vi "UHR-Fleezers Control (host) - 12.1.vi"() -> ()   [LabVIEW 2012] (continued)
                n291 = Divide "Y half step offset"(x=w520, y=2.0) -> (x/y=w534:dbl)
                n292 = Divide "X pix/step"(x=w522, y=w525) -> (x/y=w531:dbl)
                n293 = Negate(x=w534) -> (-x=w535:dbl)
                n294 = local read "Initial Y"() -> (w541:dbl)
                n295 = Multiply(x=w523, y=w532) -> (x*y=w542:dbl)
                n296 = Divide "X half step offset"(x=w520, y=2.0) -> (x/y=w528:dbl)
                n297 = Divide "X V/pix"(x=w520, y=w531) -> (x/y=w530:dbl)
                n298 = Multiply(x=w520, y=w525) -> (x*y=w537:dbl)
                n299 = Compound Arithmetic op=ADD(w535, w542, w541) -> (w512:dbl)
                "Pointer Y (V)" <- w512
                n300 = Multiply(x=w530, y=w524) -> (x*y=w539:dbl)
                n301 = Negate(x=w528) -> (-x=w527:dbl)
                n302 = local read "Initial X"() -> (w540:dbl)
                n303 = Negate(x=w539) -> (-x=w538:dbl)
                n304 = Compound Arithmetic op=ADD(w527, w537, w540, w538) -> (w513:dbl)
                "Pointer X (V)" <- w513
                n305 = case shown="True" "Set High F Confocal Spot (X-Y)" {
                  tunnel: w513 -> [_ w543]
                  tunnel: w512 -> [_ w544]
                  frame False {
                  }
                  frame True {
                    "Confocal Y 2 (V)" <- w544
                    "Confocal X 2 (V)" <- w543
                  }
                }
                n306 = Or(x="Set X Only", y="Set Confocal Spot (X-Y)") -> (x .or. y?=w516:bool)
                n307 = Or(x="Set Confocal Spot (X-Y)", y="Set Y Only") -> (x .or. y?=w515:bool)
                n308 = case shown="True" w516 {
                  tunnel: w513 -> [_ w545]
                  frame False {
                  }
                  frame True {
                    n309 = property on="AO2" class="Slide (strict)"("Val(Sgnl)"=w545) -> ()  [unwired: 2 in, 2 out]
                    "Confocal X 1 (V)" <- w545
                  }
                }
                n310 = case shown="True" w515 {
                  tunnel: w512 -> [_ w546]
                  frame False {
                  }
                  frame True {
                    n311 = property on="AO1" class="Slide (strict)"("Val(Sgnl)"=w546) -> ()  [unwired: 2 in, 2 out]
                    "Confocal Y 1 (V)" <- w546
                  }
                }
                n312 = local write "Set High F Confocal Spot (X-Y)"(w511) -> ()
                n313 = local write "Set Confocal Spot (X-Y)"(w511) -> ()
                n314 = local write "Set X Only"(w511) -> ()
                n315 = local write "Set Y Only"(w511) -> ()
              }
            }
          }
          frame 3 {
            n316 = local read "BD 2 Frequency 1 (MHz)"() -> (w547:dbl)
            n317 = local read "BD 1 Frequency 1 (MHz)"() -> (w548:dbl)
            n318 = local write "Manipulating Trap"(TRUE ("Manipulating Trap")) -> ()
            n319 = local write "Coords"(T7 {"Horizontal"=0, "Vertical"=0} ("Coords")) -> ()
            n320 = while {
              tunnel: w553 -> [w558]
              tunnel: w551 -> [w557]
              tunnel: w549 -> [w556]
              tunnel: w548 -> [w555]
              tunnel: w547 -> [w554]
              stop <- w559 stop-if-true
              n321 = event shown="[0] \"Pane\": Mouse Move" {
                selector: _ -> [_ _]
                dyn-events: _ -> [_ _]
                timeout: _ -> [_ _]
                tunnel: ["Force Manip Abort" w623] -> w559
                tunnel: w558 -> [w566 _]
                tunnel: w557 -> [w564 _]
                tunnel: w556 -> [w563 _]
                tunnel: w555 -> [w562 _]
                tunnel: w554 -> [w561 _]
                event Mouse Move {
                  n322 = event-data() -> ("Time"=w567:u32, "Coords"=w568:T7)  [unwired: 3 out]
                  n323 = Less?(x=w567, y=w566) -> (x < y?=w565:bool)
                  n324 = case "Makes sure old motion events prior to mouse click aren't used" shown="False" w565 {
                    tunnel: w568 -> [w610 _]
                    tunnel: w564 -> [w611 _]
                    tunnel: w563 -> [w588 _]
                    tunnel: w562 -> [w584 _]
                    tunnel: w561 -> [w583 _]
                    frame False {
                      n325 = Subtract(x=w610, y=w611) -> (x-y=w609:T7)
                      "Coords" <- w609
                      n326 = local read "Y RF Frequency Limits (MHz)"() -> (w569:T15)
                      n327 = To Double Precision Float(number=w609) -> (double precision float=w608:cluster{"Horizontal":dbl, "Vertical":dbl})
                      n328 = Multiply(x=cluster{"Horizontal":dbl, "Vertical":dbl} {"Horizontal"=-1.0, "Vertical"=1.0}, y="Manipulation Scaling") -> (x*y=w604:cluster{"Horizontal":dbl, "Vertical":dbl})
                      n329 = local read "X RF Frequency Limits (MHz)"() -> (w570:T15)
                      n330 = Multiply(x=w608, y=w604) -> (x*y=w606:cluster{"Horizontal":dbl, "Vertical":dbl})
                      n331 = Unbundle By Name(w606) -> ("Horizontal"=w601:dbl, "Vertical"=w605:dbl)
                      n332 = Unbundle By Name(w569) -> ("Maximum"=w572:dbl, "Minimum"=w571:dbl)
                      n333 = Boolean To (0,1)(Boolean="Manip. X?") -> (0, 1=w599:i16)
                      n334 = Boolean To (0,1)(Boolean="Manip. Y?") -> (0, 1=w596:i16)
                      n335 = local read "BD 1 Frequency 2 (MHz)"() -> (w586:dbl)
                      n336 = Multiply(x=w605, y=w596) -> (x*y=w598:dbl)
                      n337 = Multiply(x=w599, y=w601) -> (x*y=w602:dbl)
                      n338 = local read "BD 2 Frequency 2 (MHz)"() -> (w585:dbl)
                      n339 = Unbundle By Name(w570) -> ("Maximum"=w574:dbl, "Minimum"=w573:dbl)
                      n340 = Add(x=w583, y=w598) -> (x+y=w576:dbl)
                      n341 = Add(x=w584, y=w602) -> (x+y=w578:dbl)
                      n342 = In Range and Coerce(upper limit=w574, x=w578, lower limit=w573) -> (coerced(x)=w577:dbl)  [unwired: 1 out]
                      n343 = In Range and Coerce(upper limit=w572, x=w576, lower limit=w571) -> (coerced(x)=w575:dbl)  [unwired: 1 out]
                      n344 = Subtract(x=w577, y=w586) -> (x-y=w595:dbl)
                      n345 = Subtract(x=w575, y=w585) -> (x-y=w594:dbl)
                      n346 = Square(x=w595) -> (x^2=w593:dbl)
                      n347 = Square(x=w594) -> (x^2=w592:dbl)
                      n348 = Add(x=w593, y=w592) -> (x+y=w591:dbl)
                      n349 = Square Root(x=w591) -> (sqrt(x)=w587:dbl)
                      n350 = In Range and Coerce(upper limit="Limit Max (MHz)", x=w587, lower limit="Limit Min (MHz)") -> (In Range?=w580:bool)  [unwired: 1 out]
                      n351 = Not(x="Limits Enable") -> (.not. x?=w579:bool)
                      n352 = Or(x=w580, y=w579) -> (x .or. y?=w581:bool)
                      n353 = case shown="True" w581 {
                        tunnel: w588 -> [_ w621]
                        tunnel: w587 -> [_ w612]
                        tunnel: w577 -> [_ w619]
                        tunnel: w586 -> [_ w618]
                        tunnel: w575 -> [_ w617]
                        tunnel: w585 -> [_ w616]
                        tunnel: w570 -> [_ w614]
                        tunnel: w569 -> [_ w613]
                        frame False {
                        }
                        frame True {
                          n354 = local read "BD 1 Frequency 3 (MHz)"() -> (w620:dbl)
                          n355 = local read "BD 2 Frequency 3 (MHz)"() -> (w615:dbl)
                          n356 = local write "Trap Delta (MHz)"(w612) -> ()
                          n357 = call "set RF board frequency - interlace.vi"("Board 2 Frequency Limits"=w613, "Board 1 Frequency Limits"=w614, "FPGA VI Reference In"=w621, "Board 2 Frequency 3 (MHz)"=w615, "Board 1 Frequency 3 (MHz)"=w620, "Board 2 Frequency 2 (MHz)"=w616, "Board 2 Frequency 1 (MHz)"=w617, "Board 1 Frequency 2 (MHz)"=w618, "Board 1 Frequency 1  (MHz)"=w619) -> ()  [unwired: 1 in, 2 out]
                          n358 = local write "BD 2 Frequency 1 (MHz)"(w617) -> ()
                          n359 = local write "BD 1 Frequency 1 (MHz)"(w619) -> ()
                        }
                      }
                    }
                    frame True {
                    }
                  }
                }
                event Mouse Up {
                  n360 = event-data() -> ("Button"=w622:u16)  [unwired: 8 out]
                  n361 = case shown="3" w622 {
                    tunnel: [FALSE TRUE] -> w623
                    frame 0, Default {
                    }
                    frame 3 {
                      n362 = local read "Trap Delta (MHz)"() -> (w625:dbl)
                      n363 = property on="Initial delta (MHz)" class="DigNum (strict)"("Val(Sgnl)"=w625) -> ()  [unwired: 2 in, 2 out]
                      n364 = local write "Manipulating Trap"(FALSE ("Manipulating Trap")) -> ()
                    }
                  }
                }
              }
            }
          }
        }
      }
      event Mouse Move {
        n365 = event-data() -> ()  [unwired: 6 out]
      }
    }
    n366 = local read "Stop All"() -> (w441:bool)
    n367 = node-c288() -> ()  [unwired: 2 out]
  }
  n368 = timed-loop "Run Scripts, including: stage motion" {
    tunnel: w108 -> [w634]
    tunnel: w107 -> [w635]
    tunnel: [w635] -> w106
    tunnel: [w634] -> w105
    timing: w103 -> [_]
    timing-out: [_] -> w102
    tunnel: w88 -> [w633]
    tunnel: w89 -> [w632]
    tunnel: w32 -> [w629]
    tunnel: w31 -> [w628]
    tunnel: w30 -> [w630]
    tunnel: w29 -> [w631]
    stop <- w636 stop-if-true
    n369 = node-c288() -> ()  [unwired: 1 in, 1 out]
    n370 = event shown="[1] \"Move to Position\": Value Change" {
      selector: _ -> [_ _ _ _ _ _ _ _ _ _ _ _ _ _ _ _ _ _ _]
      dyn-events: _ -> [_ _ _ _ _ _ _ _ _ _ _ _ _ _ _ _ _ _ _]
      timeout: _ -> [_ _ _ _ _ _ _ _ _ _ _ _ _ _ _ _ _ _ _]
      tunnel: ["Set Position" "Move to Position" _ _ "Read Harvard" _ _ _ _ _ _ "Got ADig bead" "Force FB Data\nScript" _ "Got DNA bead" "Take Stepping Data" _ "Take Detection Laser\nImage" _] -> _
      tunnel: [_ _ _ _ _ _ _ _ _ _ _ _ _ _ _ _ _ _ w1253] -> w636
      tunnel: w634 -> [w654 w662 w675 w705 _ w750 w790 w871 w900 w1032 w1058 _ w1094 _ _ _ _ _ _]
      tunnel: w635 -> [w655 w663 w676 w706 _ w751 w791 w872 w901 w1033 w1059 _ w1095 _ _ _ _ _ _]
      tunnel: w633 -> [_ _ _ _ w735 _ _ _ _ _ _ _ _ _ _ _ _ _ _]
      tunnel: w632 -> [_ _ _ _ w734 _ _ _ _ _ _ _ _ _ _ _ _ _ _]
      tunnel: w631 -> [_ _ _ _ _ _ _ _ _ _ _ _ _ _ _ _ _ _ _]
      tunnel: w630 -> [_ _ _ _ _ _ _ _ _ _ _ _ _ _ _ _ _ _ _]
      tunnel: w629 -> [_ _ _ _ _ _ _ _ _ _ _ _ _ _ _ _ _ _ _]
      tunnel: w628 -> [_ _ _ _ _ _ _ _ _ _ _ _ _ _ _ _ _ _ _]
      event "Set Position", "Set Position 2", "Set Position 3", "Set Position 4", "Set Position 5", "Set Position 1": Value Change {
        n371 = event-data() -> ()  [unwired: 1 in, 5 out]
        n372 = Build Array("Set Position 1", "Set Position 2", "Set Position 3", "Set Position 4", "Set Position 5") -> (w653:bool[])
        n373 = Boolean Array To Number(Boolean array=w653) -> (number=w652:u32)
        n374 = Logarithm Base 2(1:w652) -> (0:w644:dbl)
        n375 = call "Read Stage Position.vi"("error in"=w654, "VISA resource name in"=w655) -> ("Current Position"=w659:cluster{dbl, dbl, dbl}, "error out"=w658:errorcluster)  [unwired: 2 out]
        n376 = Decrement(x="Position") -> (x-1=w642:dbl)
        n377 = Greater Or Equal?(x=w644, y=0.0) -> (x >= y?=w645:bool)
        n378 = Cluster To Array(cluster=w659) -> (array=w656:dbl[])
        n379 = local write "Stage Control Serial Error"(w658) -> ()
        n380 = Select(t=w644, s=w645, f=w642) -> (s? t:f=w641:dbl)
        n381 = Increment(x=w641) -> (x+1=w640:dbl)
        n382 = Build Array (concatenate)(w640, w656) -> (w639:dbl[])
        n383 = Replace Array Subset(array="Saved Stage Positions", new element=w639, index (row)=w641) -> (w657:dbl[][])  [unwired: 1 in]
        n384 = local write "Saved Stage Positions"(w657) -> ()
      }
      event "Move to Position": Value Change {
        n385 = event-data() -> ()  [unwired: 1 in, 5 out]
        n386 = flat-sequence {
          tunnel: w663 -> [w667]
          tunnel: w662 -> [w666]
          frame #0 {
            n387 = local read "Saved Stage Positions"() -> (w669:dbl[][])
            n388 = local read "Position"() -> (w668:dbl)
            n389 = local write "Stage Moving"(TRUE ("Stage Moving")) -> ()
            n390 = call "move to saved stage position.vi"("error in"=w666, "Stage VISA resource name in"=w667, "Position"=w668, "Saved Stage Positions"=w669) -> ("error out"=w665:errorcluster)  [unwired: 1 out]
            n391 = local write "Stage Control Serial Error"(w665) -> ()
          }
          frame #1 {
            n392 = call <vilib>:"Beep.vi"() -> ()  [unwired: 3 in, 9 out]
            n393 = local write "Stage Moving"(FALSE ("Stage Moving")) -> ()
          }
        }
      }
      event "Move Cap. 1 (DNA Bottom)": Value Change {
        n394 = event-data() -> ()  [unwired: 1 in, 5 out]
        n395 = local write "Move Cap. 1 (DNA Bottom)"(FALSE ("Move Cap. 1 (DNA Right)")) -> ()
        n396 = flat-sequence {
          tunnel: w675 -> [w678]
          tunnel: w676 -> [w679]
          tunnel: [w679] -> w673
          tunnel: [w678] -> w672
          tunnel: w673 -> [w681]
          tunnel: w672 -> [w680]
          frame #0 {
            n397 = property on="Sample Channel\nFlow" class="Bool (strict)"("Val(Sgnl)"="Cap 1 Samp Flow ON") -> ()  [unwired: 2 in, 2 out]
          }
          frame #1 {
            n398 = local read "Saved Stage Positions"() -> (w691:dbl[][])
            n399 = local write "Stage Moving"(TRUE ("Stage Moving")) -> ()
            n400 = Array Subset(array=w691, index (row)=0 ("index"), length (row)=1 ("length"), index (col)=1 ("index"), length (col)=3 ("length")) -> (w688:dbl[][])
            n401 = Reshape Array(w688, 3 ("dimension size")) -> (w686:dbl[])
            n402 = Array To Cluster(array=w686) -> (cluster=w685:cluster{"[0]":dbl, "[1]":dbl, "[2]":dbl})
            n403 = call "Set Stage Position.vi"("Position"=w685, "error in"=w680, "VISA resource name in"=w681) -> ("error out"=w684:errorcluster)  [unwired: 2 out]
            n404 = local write "Stage Control Serial Error"(w684) -> ()
          }
          frame #2 {
            n405 = local write "Stage Moving"(FALSE ("Stage Moving")) -> ()
            n406 = case shown="True" "Cap 1 Flow ON" {
              frame False {
              }
              frame True {
                n407 = property on="Inject Pump 1" class="Bool (strict)"("Val(Sgnl)"=TRUE ("Value (Signaling)")) -> ()  [unwired: 2 in, 2 out]
              }
            }
            n408 = call <vilib>:"Beep.vi"() -> ()  [unwired: 3 in, 9 out]
          }
          frame #3 {
            n409 = property on="Sample Channel\nFlow" class="Bool (strict)"("Val(Sgnl)"=FALSE ("Value (Signaling)")) -> ()  [unwired: 2 in, 2 out]
            n410 = local read "Cap. 2 BD T1?\n(ADig T1, DNA T2)"() -> (w698:bool)
            n411 = case shown="True" w698 {
              tunnel: "Cap 1 T ON" -> [w700 w701]
              frame False {
                n412 = property on="Trap 1 (ON/OFF)" class="Bool (strict)"("Val(Sgnl)"=w700) -> ()  [unwired: 2 in, 2 out]
              }
              frame True {
                n413 = property on="Trap 2 (ON/OFF)" class="Bool (strict)"("Val(Sgnl)"=w701) -> ()  [unwired: 2 in, 2 out]
              }
            }
            n414 = property on="Got DNA bead" class="Bool"("Key Focus"=TRUE) -> ()  [unwired: 2 in, 2 out]
          }
        }
      }
      event "Move Cap. 2 (ADig Top)": Value Change {
        n415 = event-data() -> ()  [unwired: 1 in, 5 out]
        n416 = local write "Move Cap. 2 (ADig Top)"(FALSE ("Move Cap. 2 (ADig Left)")) -> ()
        n417 = flat-sequence {
          tunnel: w705 -> [w708]
          tunnel: w706 -> [w709]
          tunnel: [w709] -> w703
          tunnel: [w708] -> w702
          tunnel: w703 -> [w712]
          tunnel: w702 -> [w711]
          frame #0 {
            n418 = property on="Sample Channel\nFlow" class="Bool (strict)"("Val(Sgnl)"="Cap 2 Samp Flow ON") -> ()  [unwired: 2 in, 2 out]
          }
          frame #1 {
            w710 = FALSE ("Value (Signaling)")
            n419 = local read "Saved Stage Positions"() -> (w722:dbl[][])
            n420 = local write "Stage Moving"(TRUE ("Stage Moving")) -> ()
            n421 = Array Subset(array=w722, index (row)=1 ("index"), length (row)=1 ("length"), index (col)=1 ("index"), length (col)=3 ("length")) -> (w719:dbl[][])
            n422 = Reshape Array(w719, 3 ("dimension size")) -> (w717:dbl[])
            n423 = property on="Trap 1 (ON/OFF)" class="Bool (strict)"("Val(Sgnl)"=w710) -> ()  [unwired: 2 in, 2 out]
            n424 = property on="Trap 1 (ON/OFF)" class="Bool (strict)"("Val(Sgnl)"=w710) -> ()  [unwired: 2 in, 2 out]
            n425 = Array To Cluster(array=w717) -> (cluster=w716:cluster{"[0]":dbl, "[1]":dbl, "[2]":dbl})
            n426 = call "Set Stage Position.vi"("Position"=w716, "error in"=w711, "VISA resource name in"=w712) -> ("error out"=w715:errorcluster)  [unwired: 2 out]
            n427 = local write "Stage Control Serial Error"(w715) -> ()
          }
          frame #2 {
            n428 = local write "Stage Moving"(FALSE ("Stage Moving")) -> ()
            n429 = call <vilib>:"Beep.vi"() -> ()  [unwired: 3 in, 9 out]
            n430 = case shown="True" "Cap 2 Flow ON" {
              frame False {
              }
              frame True {
                n431 = property on="Inject Pump 3" class="Bool (strict)"("Val(Sgnl)"=TRUE ("Value (Signaling)")) -> ()  [unwired: 2 in, 2 out]
              }
            }
          }
          frame #3 {
            n432 = property on="Sample Channel\nFlow" class="Bool (strict)"("Val(Sgnl)"=FALSE ("Value (Signaling)")) -> ()  [unwired: 2 in, 2 out]
            n433 = case shown="False" "Cap. 2 BD T1?\n(ADig T1, DNA T2)" {
              tunnel: "Cap 2 T ON" -> [w731 w732]
              frame False {
                n434 = property on="Trap 2 (ON/OFF)" class="Bool (strict)"("Val(Sgnl)"=w731) -> ()  [unwired: 2 in, 2 out]
              }
              frame True {
                n435 = property on="Trap 1 (ON/OFF)" class="Bool (strict)"("Val(Sgnl)"=w732) -> ()  [unwired: 2 in, 2 out]
              }
            }
            n436 = property on="Got ADig bead" class="Bool"("Key Focus"=TRUE) -> ()  [unwired: 2 in, 2 out]
          }
        }
      }
      event "Read Harvard": Value Change {
        n437 = event-data() -> ()  [unwired: 1 in, 5 out]
        n438 = Concatenate Strings("write buffer", "\r") -> (w737:string)
        n439 = VISA Write(VISA resource name=w735, write buffer=w737, error in (no error)=w734) -> (VISA resource name out=w746:refnum<visa-resource-name>, error out=w745:errorcluster)  [unwired: 1 out]
        n440 = stacked-sequence {
          tunnel: [w749] -> w744
          tunnel: w746 -> [w749]
          tunnel: w745 -> [w748]
          tunnel: [w748] -> w739
          frame #0 {
            n441 = Wait (ms)(milliseconds to wait=50) -> ()  [unwired: 1 out]
          }
        }
        n442 = property class="Instr"(reference=w744, error in=w739) -> (reference out=w743:refnum<visa-resource-name>, error out=w741:errorcluster, "Serial Settings:Number of Bytes at Serial Port"=w742:u32)
        "Serial Settings:Number of Bytes at Serial Port" <- w742
        n443 = VISA Read(VISA resource name=w743, byte count=w742, error in (no error)=w741) -> (read buffer=w740:string)  [unwired: 3 out]
        "read buffer" <- w740
        n444 = Fract/Exp String To Number(string=w740) -> ()  [unwired: 5 out]
      }
      event "+z", "-z": Value Change {
        n445 = event-data() -> ()  [unwired: 1 in, 5 out]
        n446 = flat-sequence {
          tunnel: w750 -> [w772]
          tunnel: w751 -> [w752]
          frame #0 {
            n447 = call "Read Stage Position.vi"("error in"=w772, "VISA resource name in"=w752) -> ("Current Position"=w757:cluster{dbl, dbl, dbl}, "error out"=w770:errorcluster, "VISA resource name out"=w771:refnum<visa-resource-name>)  [unwired: 1 out]
            n448 = local read "Saved Stage Positions"() -> (w781:dbl[][])
            n449 = Divide(x="z nudge increment (um)", y=1000.0) -> (x/y=w769:dbl)
            n450 = Boolean To (0,1)(Boolean="+z") -> (0, 1=w761:i16)
            n451 = Boolean To (0,1)(Boolean="-z") -> (0, 1=w762:i16)
            n452 = Array Subset(array=w781, index (row)=1 ("index"), length (row)=1 ("length"), index (col)=1 ("index"), length (col)=3 ("length")) -> (w778:dbl[][])
            n453 = Multiply(x=w761, y=w769) -> (x*y=w765:dbl)
            n454 = Multiply(x=w762, y=w769) -> (x*y=w763:dbl)
            n455 = Unbundle(w757) -> (w755:dbl, w754:dbl, w758:dbl)
            n456 = Negate(x=w763) -> (-x=w764:dbl)
            n457 = Reshape Array(w778, 3 ("dimension size")) -> (w776:dbl[])
            n458 = Add(x=w765, y=w764) -> (x+y=w766:dbl)
            n459 = Array To Cluster(array=w776) -> ()  [unwired: 1 out]
            n460 = Add(x=w766, y=w758) -> (x+y=w756:dbl)
            n461 = Bundle(cluster=w757, w755, w754, w756) -> (w753:cluster{dbl, dbl, dbl})
            n462 = call "Set Stage Position.vi"("Position"=w753, "error in"=w770, "VISA resource name in"=w771) -> ("error out"=w775:errorcluster)  [unwired: 2 out]
            n463 = local write "Stage Moving"(TRUE ("Stage Moving")) -> ()
            n464 = local write "Stage Control Serial Error"(w775) -> ()
          }
          frame #1 {
            n465 = local write "Stage Moving"(FALSE ("Stage Moving")) -> ()
            n466 = call <vilib>:"Beep.vi"() -> ()  [unwired: 3 in, 9 out]
          }
        }
      }
      event "Cal/Data Acq. Spot": Value Change {
        n467 = event-data() -> ()  [unwired: 1 in, 5 out]
        n468 = flat-sequence {
          tunnel: w790 -> [w794]
          tunnel: w791 -> [w795]
          tunnel: [w795] -> w787
          tunnel: [w794] -> w786
          tunnel: w787 -> [w800]
          tunnel: w786 -> [w799]
          tunnel: ["Cal @ (MHz)"] -> w784
          tunnel: [w804] -> w788
          tunnel: w784 -> [w804]
          tunnel: w788 -> [w813]
          tunnel: ["W/ Offset 1"] -> w785
          tunnel: w788 -> [w834]
          tunnel: w785 -> [w832]
          frame #0 {
            n469 = property on="Sample Channel\nFlow" class="Bool (strict)"("Val(Sgnl)"="Daq spot flow on") -> ()  [unwired: 2 in, 2 out]
            n470 = Wait (ms)(milliseconds to wait=u32 250) -> ()  [unwired: 1 out]
          }
          frame #1 {
            n471 = local read "Saved Stage Positions"() -> (w797:dbl[][])
            n472 = property on="Trap Delta (MHz)" class="DigNum (strict)"("Val(Sgnl)"="Cal @ (MHz)") -> ()  [unwired: 2 in, 2 out]
            n473 = local write "Stage Moving"(TRUE ("Stage Moving")) -> ()
            n474 = call "move to saved stage position.vi"("error in"=w799, "Stage VISA resource name in"=w800, "Position"="Cal Stage Position", "Saved Stage Positions"=w797) -> ("error out"=w798:errorcluster)  [unwired: 1 out]
            n475 = local write "Stage Control Serial Error"(w798) -> ()
          }
          frame #2 {
            n476 = local write "Stage Moving"(FALSE ("Stage Moving")) -> ()
            n477 = property on="Sample Channel\nFlow" class="Bool (strict)"("Val(Sgnl)"="Flow ON during cal?") -> ()  [unwired: 2 in, 2 out]
            n478 = call <vilib>:"Beep.vi"() -> ()  [unwired: 3 in, 9 out]
          }
          frame #3 {
            n479 = Wait (ms)(milliseconds to wait=u32 1000) -> ()  [unwired: 1 out]
          }
          frame #4 {
            n480 = property on="Save Calibration" class="Bool (strict)"("Val(Sgnl)"=TRUE ("Value (Signaling)")) -> ()  [unwired: 2 in, 2 out]
          }
          frame #5 {
            n481 = Wait (ms)(milliseconds to wait=u32 2000) -> ()  [unwired: 1 out]
          }
          frame #6 {
            # "Check to see if \nsaving done"
            n482 = while {
              stop <- w809 stop-if-true
              n483 = local read "Saving..."() -> (w810:bool)
              n484 = Wait (ms)(milliseconds to wait=u32 100) -> ()  [unwired: 1 out]
              n485 = Not(x=w810) -> (.not. x?=w809:bool)
            }
          }
          frame #7 {
            n486 = case shown="True" "W/ Offset 1" {
              tunnel: w813 -> [_ w814]
              frame False {
              }
              frame True {
                n487 = stacked-sequence {
                  tunnel: w814 -> [_ _ _ _ _ _ _ w831]
                  frame #0 {
                    n488 = property on="Trap Delta (MHz)" class="DigNum (strict)"("Val(Sgnl)"="Offset 1 Start (MHz)") -> ()  [unwired: 2 in, 2 out]
                    n489 = Replace Array Subset(array=u32[] [0] ("Index Values"), new element="Offset 1 Set", index=0) -> (w815:u32[])
                    n490 = property on="Saved AOD Raster Scan Parameter Sets" class="Arr (strict)"("Index Values"=w815) -> ()  [unwired: 2 in, 2 out]
                  }
                  frame #1 {
                    n491 = Wait (ms)(milliseconds to wait=u32 200) -> ()  [unwired: 1 out]
                  }
                  frame #2 {
                    n492 = property on="Load parameters" class="Bool (strict)"("Val(Sgnl)"=TRUE ("Value (Signaling)")) -> ()  [unwired: 2 in, 2 out]
                  }
                  frame #3 {
                    n493 = Wait (ms)(milliseconds to wait=u32 200) -> ()  [unwired: 1 out]
                  }
                  frame #4 {
                    n494 = property on="Trap Raster Scan" class="Bool (strict)"("Val(Sgnl)"=TRUE ("Value (Signaling)")) -> ()  [unwired: 2 in, 2 out]
                  }
                  frame #5 {
                    n495 = Wait (ms)(milliseconds to wait=u32 2000) -> ()  [unwired: 1 out]
                  }
                  frame #6 {
                    n496 = while {
                      stop <- w828 stop-if-true
                      n497 = local read "Raster Scanning..."() -> (w830:bool)
                      n498 = local read "Saving..."() -> (w826:bool)
                      n499 = Wait (ms)(milliseconds to wait=u32 100) -> ()  [unwired: 1 out]
                      n500 = Not(x=w826) -> (.not. x?=w825:bool)
                      n501 = Not(x=w830) -> (.not. x?=w827:bool)
                      n502 = And(x=w827, y=w825) -> (x .and. y?=w828:bool)
                    }
                  }
                  frame #7 {
                    n503 = property on="Trap Delta (MHz)" class="DigNum (strict)"("Val(Sgnl)"=w831) -> ()  [unwired: 2 in, 2 out]
                  }
                }
              }
            }
          }
          frame #8 {
            n504 = local read "Save ave N"() -> (w833:dbl)
            n505 = case shown="False" "W/ Offset 2" {
              tunnel: w834 -> [_ w841]
              tunnel: w833 -> [_ w840]
              tunnel: w832 -> [w836 _]
              frame False {
                n506 = case shown="False" w836 {
                  frame False {
                    n507 = Multiply(x="Cal read wait (s)", y=u32 1000 ("milliseconds to wait")) -> (x*y=w838:u32)
                    n508 = Wait (ms)(milliseconds to wait=w838) -> ()  [unwired: 1 out]
                  }
                  frame True {
                  }
                }
              }
              frame True {
                n509 = stacked-sequence {
                  tunnel: w841 -> [_ _ _ _ _ _ _ _ _ w862 _ _]
                  tunnel: w840 -> [_ _ _ _ _ _ _ _ _ w860 _ _]
                  frame #0 {
                    n510 = property on="Save ave N" class="DigNum (strict)"("Val(Sgnl)"=1.0 ("Value (Signaling)")) -> ()  [unwired: 2 in, 2 out]
                  }
                  frame #1 {
                    n511 = Wait (ms)(milliseconds to wait=u32 500) -> ()  [unwired: 1 out]
                  }
                  frame #2 {
                    n512 = property on="Trap Delta (MHz)" class="DigNum (strict)"("Val(Sgnl)"="Offset 2 Start (MHz)") -> ()  [unwired: 2 in, 2 out]
                    n513 = Replace Array Subset(array=u32[] [0] ("Index Values"), new element="Offset 2 Set", index=0) -> (w846:u32[])
                    n514 = property on="Saved AOD Raster Scan Parameter Sets" class="Arr (strict)"("Index Values"=w846) -> ()  [unwired: 2 in, 2 out]
                  }
                  frame #3 {
                    n515 = Wait (ms)(milliseconds to wait=u32 500) -> ()  [unwired: 1 out]
                  }
                  frame #4 {
                    n516 = property on="Load parameters" class="Bool (strict)"("Val(Sgnl)"=TRUE ("Value (Signaling)")) -> ()  [unwired: 2 in, 2 out]
                  }
                  frame #5 {
                    n517 = Wait (ms)(milliseconds to wait=u32 500) -> ()  [unwired: 1 out]
                  }
                  frame #6 {
                    n518 = property on="Trap Raster Scan" class="Bool (strict)"("Val(Sgnl)"=TRUE ("Value (Signaling)")) -> ()  [unwired: 2 in, 2 out]
                  }
                  frame #7 {
                    n519 = Wait (ms)(milliseconds to wait=u32 2000) -> ()  [unwired: 1 out]
                  }
                  frame #8 {
                    n520 = while {
                      stop <- w855 stop-if-true
                      n521 = local read "Raster Scanning..."() -> (w858:bool)
                      n522 = local read "Saving..."() -> (w856:bool)
                      n523 = Wait (ms)(milliseconds to wait=u32 100) -> ()  [unwired: 1 out]
                      n524 = Not(x=w856) -> (.not. x?=w854:bool)
                      n525 = Not(x=w858) -> (.not. x?=w857:bool)
                      n526 = And(x=w857, y=w854) -> (x .and. y?=w855:bool)
                    }
                  }
                  frame #9 {
                    n527 = property on="Trap Delta (MHz)" class="DigNum (strict)"("Val(Sgnl)"=w862) -> ()  [unwired: 2 in, 2 out]
                    n528 = property on="Saved AOD Raster Scan Parameter Sets" class="Arr (strict)"("Index Values"=u32[] [0]) -> ()  [unwired: 2 in, 2 out]
                    n529 = property on="Save ave N" class="DigNum (strict)"("Val(Sgnl)"=w860) -> ()  [unwired: 2 in, 2 out]
                  }
                  frame #10 {
                    n530 = Wait (ms)(milliseconds to wait=u32 500) -> ()  [unwired: 1 out]
                  }
                  frame #11 {
                    n531 = property on="Load parameters" class="Bool (strict)"("Val(Sgnl)"=TRUE ("Value (Signaling)")) -> ()  [unwired: 2 in, 2 out]
                  }
                }
              }
            }
          }
          frame #9 {
            n532 = property on="Read Cal" class="Bool (strict)"("Val(Sgnl)"=TRUE ("Value (Signaling)")) -> ()  [unwired: 2 in, 2 out]
          }
          frame #10 {
            n533 = Wait (ms)(milliseconds to wait=u32 1000) -> ()  [unwired: 1 out]
          }
          frame #11 {
            n534 = property on="Fish for Tether" class="Bool (strict)"("Val(Sgnl)"=TRUE ("Value (Signaling)")) -> ()  [unwired: 2 in, 2 out]
          }
        }
        n535 = local write "Cal/Data Acq. Spot"(FALSE ("Cal/Data Acq. Spot")) -> ()
      }
      event "Dump Beads": Value Change {
        n536 = event-data() -> ()  [unwired: 1 in, 5 out]
        n537 = flat-sequence {
          tunnel: ["Dump spot flow on?"] -> w868
          tunnel: [w879] -> w869
          tunnel: w868 -> [w879]
          tunnel: w872 -> [w884]
          tunnel: w871 -> [w883]
          tunnel: [w881] -> w870
          tunnel: w869 -> [w881]
          tunnel: w870 -> [w894]
          frame #0 {
            w873 = FALSE ("Value (Signaling)")
            n538 = local read "Saving..."() -> (w875:bool)
            n539 = local write "Dump Beads"(FALSE ("Dump Beads")) -> ()
            n540 = property on="Inject Pump 3" class="Bool (strict)"("Val(Sgnl)"=w873) -> ()  [unwired: 2 in, 2 out]
            n541 = property on="Inject Pump 1" class="Bool (strict)"("Val(Sgnl)"=w873) -> ()  [unwired: 2 in, 2 out]
            n542 = local write "Stop Saving"(w875) -> ()
          }
          frame #1 {
            w876 = FALSE ("Fl. Triggered...")
            n543 = case shown="True" "Dump spot flow on?" {
              frame False {
              }
              frame True {
                n544 = property on="Sample Channel\nFlow" class="Bool (strict)"("Val(Sgnl)"=TRUE ("Stage Moving")) -> ()  [unwired: 2 in, 2 out]
              }
            }
            n545 = local write "Fl. Triggered..."(w876) -> ()
            n546 = local write "Tether"(w876) -> ()
            n547 = property on="Green Laser ON/Interlacing" class="Bool (strict)"("Val(Sgnl)"=w876) -> ()  [unwired: 2 in, 2 out]
            n548 = property on="Trap Pos. FB ON" class="Bool (strict)"("Val(Sgnl)"=w876) -> ()  [unwired: 2 in, 2 out]
            n549 = property on="Trap Trig. Fl." class="Bool (strict)"("Val(Sgnl)"=w876) -> ()  [unwired: 2 in, 2 out]
            n550 = property on="Fl. Triggered..." class="Bool (strict)"("Val(Sgnl)"=w876) -> ()  [unwired: 2 in, 2 out]
            n551 = property on="Dip for Protein" class="Bool (strict)"("Val(Sgnl)"=w876) -> ()  [unwired: 2 in, 2 out]
            n552 = property on="Pause dwell" class="Bool (strict)"("Val(Sgnl)"=w876) -> ()  [unwired: 2 in, 2 out]
          }
          frame #2 {
            n553 = property on="Trap Pos. FB Offset Factor" class="DigNum (strict)"("Val(Sgnl)"=i64 0 ("Value (Signaling)")) -> ()  [unwired: 2 in, 2 out]
          }
          frame #3 {
            n554 = local read "Saved Stage Positions"() -> (w885:dbl[][])
            n555 = local write "Stage Moving"(TRUE ("Stage Moving")) -> ()
            n556 = Array Subset(array=w885, index (row)=3 ("index"), length (row)=1 ("length"), index (col)=1 ("index"), length (col)=3 ("length")) -> (w890:dbl[][])
            n557 = Reshape Array(w890, 3 ("dimension size")) -> (w888:dbl[])
            n558 = Array To Cluster(array=w888) -> (cluster=w887:cluster{"[0]":dbl, "[1]":dbl, "[2]":dbl})
            n559 = call "Set Stage Position.vi"("Position"=w887, "error in"=w883, "VISA resource name in"=w884) -> ()  [unwired: 3 out]
          }
          frame #4 {
            w895 = FALSE ("Value (Signaling)")
            n560 = case shown="True" w894 {
              frame False {
              }
              frame True {
                n561 = property on="Sample Channel\nFlow" class="Bool (strict)"("Val(Sgnl)"=FALSE ("Stage Moving")) -> ()  [unwired: 2 in, 2 out]
              }
            }
            n562 = property on="Trap 1 (ON/OFF)" class="Bool (strict)"("Val(Sgnl)"=w895) -> ()  [unwired: 2 in, 2 out]
            n563 = property on="Trap 2 (ON/OFF)" class="Bool (strict)"("Val(Sgnl)"=w895) -> ()  [unwired: 2 in, 2 out]
            n564 = call <vilib>:"Beep.vi"() -> ()  [unwired: 3 in, 9 out]
          }
          frame #5 {
            n565 = property on="Move Cap. 2 (ADig Top)" class="Bool (strict)"("Val(Sgnl)"=TRUE ("Value (Signaling)")) -> ()  [unwired: 2 in, 2 out]
            n566 = property on="Tab Control" class="TabCtl (strict)"("Val(Sgnl)"=T4."Status" ("Value (Signaling)")) -> ()  [unwired: 2 in, 2 out]
          }
        }
      }
      event "Dip for Protein": Value Change {
        n567 = event-data() -> ()  [unwired: 1 in, 5 out]
        n568 = case shown="True" "Dip for Protein" {
          tunnel: w901 -> [_ w903]
          tunnel: w900 -> [_ w902]
          frame False {
          }
          frame True {
            n569 = while {
              tunnel: w903 -> [w914]
              tunnel: w902 -> [w913]
              i -> [w908]
              stop <- w910 stop-if-true
              n570 = Increment(x=w908) -> (x+1=→"Dip #":i32)
              n571 = flat-sequence {
                tunnel: w913 -> [w925]
                tunnel: w914 -> [w926]
                tunnel: [w926] -> w918
                tunnel: [w925] -> w917
                tunnel: [w919] -> w904
                tunnel: [w931] -> w912
                tunnel: [w932] -> w911
                tunnel: w918 -> [w933]
                tunnel: w917 -> [w934]
                tunnel: [w929] -> w905
                tunnel: w904 -> [w929]
                tunnel: [w942] -> w916
                tunnel: w912 -> [w942]
                tunnel: [w941] -> w915
                tunnel: w911 -> [w941]
                tunnel: [w938] -> w909
                tunnel: [w937] -> w906
                tunnel: w905 -> [w937]
                tunnel: w915 -> [w962]
                tunnel: w916 -> [w963]
                tunnel: w909 -> [w964]
                tunnel: w906 -> [w961]
                tunnel: [w1020] -> w910
                frame #0 {
                  n572 = local read "Trap Pos. FB ON"() -> (w919:bool)
                  n573 = Compound Arithmetic op=AND("Flow ON\nduring dip?", "FB OFF when \nflow ON", w919) -> (w920:bool)
                  n574 = case shown="True" "Move trap \nbefore dip move?" {
                    frame False {
                    }
                    frame True {
                      n575 = property on="Trap Delta (MHz)" class="DigNum (strict)"("Val(Sgnl)"="Dipping Delta (MHz)") -> ()  [unwired: 2 in, 2 out]
                    }
                  }
                  n576 = property on="Green Laser ON/Interlacing" class="Bool (strict)"("Val(Sgnl)"="Green ON\nbefore dip?") -> ()  [unwired: 2 in, 2 out]
                  n577 = property on="Sample Channel\nFlow" class="Bool (strict)"("Val(Sgnl)"="Flow ON\nduring dip?") -> ()  [unwired: 2 in, 2 out]
                  n578 = case shown="True" w920 {
                    frame False {
                    }
                    frame True {
                      n579 = property on="Trap Pos. FB ON" class="Bool (strict)"("Val(Sgnl)"=FALSE ("Value (Signaling)")) -> ()  [unwired: 2 in, 2 out]
                    }
                  }
                }
                frame #1 {
                  n580 = local read "Saved Stage Positions"() -> (w936:dbl[][])
                  n581 = local write "Cancel dwell"(FALSE ("Cancel dwell")) -> ()
                  n582 = call "move to saved stage position.vi"("error in"=w934, "Stage VISA resource name in"=w933, "Position"="Dip Stage \nPosition", "Saved Stage Positions"=w936) -> ("VISA resource name out"=w931:refnum<visa-resource-name>, "error out"=w932:errorcluster)
                }
                frame #2 {
                  n583 = node-c288() -> (w940:T20)  [unwired: 4 in]
                  n584 = timed-loop {
                    timing: w940 -> [_]
                    timing-out: [_] -> w939
                    tunnel: [w946] -> w938
                    i -> [w943]
                    stop <- w947 stop-if-true
                    n585 = node-c288() -> ()  [unwired: 1 in, 1 out]
                    n586 = Greater Or Equal?(x=w943, y="Dip Duration (s)") -> (x >= y?=w955:bool)
                    n587 = local read "Dip for Protein"() -> (w948:bool)
                    n588 = local read "Dump Beads"() -> (w945:bool)
                    n589 = local read "Cancel dwell"() -> (w954:bool)
                    n590 = local read "Pause dwell"() -> (w951:bool)
                    n591 = Not(x=w948) -> (.not. x?=w953:bool)
                    n592 = Compound Arithmetic op=OR(w954, w955, w953) -> (w952:bool)
                    n593 = Select(t=FALSE, s=w951, f=w952) -> (s? t:f=w949:bool)
                    n594 = Not(x=w945) -> (.not. x?=w944:bool)
                    n595 = node-c288() -> ()  [unwired: 1 in, 1 out]
                    n596 = And(x=w948, y=w944) -> (x .and. y?=w946:bool)
                    n597 = Or(x=w949, y=w945) -> (x .or. y?=w947:bool)
                    "Dip Time (s)" <- w943
                  }
                  n598 = node-c288(w939) -> ()  [unwired: 1 out]
                }
                frame #3 {
                  n599 = case shown="True" w964 {
                    tunnel: w963 -> [_ w969]
                    tunnel: w962 -> [_ w968]
                    tunnel: w961 -> [_ w965]
                    frame False {
                    }
                    frame True {
                      n600 = flat-sequence {
                        tunnel: w968 -> [w973]
                        tunnel: w969 -> [w974]
                        tunnel: [w974] -> w967
                        tunnel: [w973] -> w966
                        tunnel: w965 -> [w970]
                        tunnel: w967 -> [w984]
                        tunnel: w966 -> [w983]
                        tunnel: w965 -> [w992]
                        frame #0 {
                          n601 = local read "Sample Channel\nFlow"() -> (w972:bool)
                          n602 = case shown="True" w972 {
                            tunnel: "Flow ON \nduring return\nfrom dip?" -> [w975 w978]
                            tunnel: w970 -> [_ w977]
                            frame False {
                              n603 = case shown="True" w975 {
                                frame False {
                                }
                                frame True {
                                n604 = property on="Sample Channel\nFlow" class="Bool (strict)"("Val(Sgnl)"=TRUE ("Value (Signaling)")) -> ()  [unwired: 2 in, 2 out]
                                }
                              }
                            }
                            frame True {
                              n605 = case shown="False" w978 {
                                tunnel: w977 -> [w979 _]
                                frame False {
                                n606 = property on="Trap Pos. FB ON" class="Bool (strict)"("Val(Sgnl)"=w979) -> ()  [unwired: 2 in, 2 out]
                                n607 = property on="Sample Channel\nFlow" class="Bool (strict)"("Val(Sgnl)"=FALSE ("Value (Signaling)")) -> ()  [unwired: 2 in, 2 out]
                                }
                                frame True {
                                }
                              }
                            }
                          }
                        }
                        frame #1 {
                          # "For turning on green laser before stage reaches lower spot"
                          n608 = case shown="True" "Green ON\nafter start\nreturn?" {
                            frame False {
                            }
                            frame True {
                              n609 = flat-sequence {
                                frame #0 {
                                n610 = Multiply(x="Green delay after \nstart return (s)", y=1000.0) -> (x*y=w989:dbl)
                                n611 = Wait (ms)(milliseconds to wait=w989) -> ()  [unwired: 1 out]
                                }
                                frame #1 {
                                n612 = property on="Green Laser ON/Interlacing" class="Bool (strict)"("Val(Sgnl)"=TRUE ("Value (Signaling)")) -> ()  [unwired: 2 in, 2 out]
                                }
                              }
                            }
                          }
                          n613 = local read "Saved Stage Positions"() -> (w987:dbl[][])
                          n614 = local write "Cancel dwell"(FALSE ("Cancel dwell")) -> ()
                          n615 = call "move to saved stage position.vi"("error in"=w983, "Stage VISA resource name in"=w984, "Position"="Return Stage \nPosition", "Saved Stage Positions"=w987) -> ("error out"=w985:errorcluster)  [unwired: 1 out]
                          n616 = local write "Stage Control Serial Error"(w985) -> ()
                        }
                        frame #2 {
                          n617 = property on="Trap Pos. FB ON" class="Bool (strict)"("Val(Sgnl)"=w992) -> ()  [unwired: 2 in, 2 out]
                          n618 = case shown="True" "Green ON \nafter return?" {
                            frame False {
                            }
                            frame True {
                              n619 = property on="Green Laser ON/Interlacing" class="Bool (strict)"("Val(Sgnl)"=TRUE ("Value (Signaling)")) -> ()  [unwired: 2 in, 2 out]
                            }
                          }
                          n620 = case shown="True" "Move trap after return?" {
                            frame False {
                            }
                            frame True {
                              n621 = property on="Trap Delta (MHz)" class="DigNum (strict)"("Val(Sgnl)"="Dip Trap Delta 2 (MHz)") -> ()  [unwired: 2 in, 2 out]
                            }
                          }
                          n622 = case shown="True" "Save data after return?" {
                            frame False {
                            }
                            frame True {
                              n623 = property on="Start Saving" class="Bool (strict)"("Val(Sgnl)"=TRUE ("Value (Signaling)")) -> ()  [unwired: 2 in, 2 out]
                            }
                          }
                          n624 = property on="Sample Channel\nFlow" class="Bool (strict)"("Val(Sgnl)"="Flow ON\nduring daq?") -> ()  [unwired: 2 in, 2 out]
                        }
                        frame #3 {
                          n625 = node-c288() -> (w1001:T20)  [unwired: 4 in]
                          n626 = timed-loop {
                            timing: w1001 -> [_]
                            timing-out: [_] -> w1000
                            i -> [w1002]
                            stop <- w1004 stop-if-true
                            n627 = node-c288() -> ()  [unwired: 1 in, 1 out]
                            n628 = local read "Dump Beads"() -> (w1003:bool)
                            n629 = Greater Or Equal?(x=w1002, y="Dwell Duration (s)") -> (x >= y?=w1009:bool)
                            n630 = local read "Dip for Protein"() -> (w1006:bool)
                            n631 = Not(x=w1006) -> (.not. x?=w1005:bool)
                            n632 = Compound Arithmetic op=OR(w1009, "Cancel dwell", w1005) -> (w1008:bool)
                            n633 = node-c288() -> ()  [unwired: 1 in, 1 out]
                            n634 = Select(t=FALSE, s="Pause dwell", f=w1008) -> (s? t:f=w1011:bool)
                            n635 = Or(x=w1011, y=w1003) -> (x .or. y?=w1004:bool)
                            "Dwell Time (s)" <- w1002
                          }
                          n636 = node-c288(w1000) -> ()  [unwired: 1 out]
                        }
                      }
                    }
                  }
                }
                frame #4 {
                  n637 = local read "Dip for Protein"() -> (w1021:bool)
                  n638 = local read "Dump Beads"() -> (w1018:bool)
                  n639 = local write "Cancel dwell"(FALSE ("Cancel dwell")) -> ()
                  n640 = Not(x=w1021) -> (.not. x?=w1022:bool)
                  n641 = Not(x="Cont. Repeat Dipping?") -> (.not. x?=w1024:bool)
                  n642 = Compound Arithmetic op=OR(w1022, w1024, w1018) -> (w1020:bool)
                }
              }
            }
          }
        }
      }
      event "Profile": Value Change {
        n643 = event-data() -> ()  [unwired: 1 in, 5 out]
        n644 = flat-sequence {
          tunnel: w1033 -> [w1036]
          tunnel: w1032 -> [w1044]
          tunnel: [w1038] -> w1031
          tunnel: [w1037] -> w1030
          tunnel: [w1035] -> w1028
          tunnel: [w1034] -> w1025
          tunnel: w1031 -> [w1051]
          tunnel: w1030 -> [w1050]
          tunnel: [w1048] -> w1029
          tunnel: w1028 -> [w1049]
          tunnel: [w1047] -> w1027
          tunnel: [w1046] -> w1026
          tunnel: w1025 -> [w1046]
          tunnel: w1029 -> [w1055]
          tunnel: w1027 -> [w1054]
          tunnel: w1026 -> [w1053]
          frame #0 {
            n645 = call "Read Stage Position.vi"("error in"=w1044, "VISA resource name in"=w1036) -> ("Current Position"=w1034:cluster{dbl, dbl, dbl}, "error out"=w1037:errorcluster, "VISA resource name out"=w1035:refnum<visa-resource-name>)  [unwired: 1 out]
            "Current Position" <- w1034
            n646 = local write "Stage Control Serial Error"(w1037) -> ()
            n647 = Unbundle(w1034) -> (w1041:dbl, w1043:dbl, w1039:dbl)
            n648 = Add(x=w1043, y="Y change (mm)") -> (x+y=w1040:dbl)
            n649 = Bundle(w1041, w1040, w1039) -> (w1038:cluster{dbl, dbl, dbl})  [unwired: 1 in]
          }
          frame #1 {
            # "move to new position and start saving"
            n650 = local write "Stage Moving"(TRUE ("Stage Moving")) -> ()
            n651 = local write "Start Saving"(TRUE ("Start Saving")) -> ()
            n652 = call "Set Stage Position.vi"("Position"=w1051, "error in"=w1050, "VISA resource name in"=w1049) -> ("error out"=w1047:errorcluster, "VISA resource name out"=w1048:refnum<visa-resource-name>)  [unwired: 1 out]
          }
          frame #2 {
            # "go back to start"
            n653 = call "Set Stage Position.vi"("Position"=w1053, "error in"=w1054, "VISA resource name in"=w1055) -> ()  [unwired: 3 out]
          }
          frame #3 {
            # "stop saving"
            n654 = local write "Stop Saving"(TRUE ("Stop Saving")) -> ()
            n655 = local write "Stage Moving"(FALSE ("Stage Moving")) -> ()
          }
        }
      }
      event "Move to Position 1", "Move to Position 2", "Move to Position 3", "Move to Position 4", "Move to Position 5", "Lower Ch. Cap.": Value Change {
        n656 = event-data() -> ()  [unwired: 1 in, 5 out]
        n657 = Or(x="Move to Position 5", y="Lower Ch. Cap.") -> (x .or. y?=w1061:bool)
        n658 = Build Array("Move to Position 1", "Move to Position 2", "Move to Position 3", "Move to Position 4", w1061) -> (w1064:bool[])
        n659 = Boolean Array To Number(Boolean array=w1064) -> (number=w1063:u32)
        n660 = Logarithm Base 2(1:w1063) -> (0:w1062:dbl)
        n661 = flat-sequence {
          tunnel: w1062 -> [w1073]
          tunnel: w1059 -> [w1071]
          tunnel: w1058 -> [w1070]
          frame #0 {
            n662 = local read "Saved Stage Positions"() -> (w1081:dbl[][])
            n663 = Array Subset(array=w1081, index (row)=w1073, length (row)=1 ("length"), index (col)=1 ("index"), length (col)=3 ("length")) -> (w1078:dbl[][])
            n664 = Reshape Array(w1078, 3 ("dimension size")) -> (w1076:dbl[])
            n665 = Array To Cluster(array=w1076) -> (cluster=w1075:cluster{"[0]":dbl, "[1]":dbl, "[2]":dbl})
            n666 = call "Set Stage Position.vi"("Position"=w1075, "error in"=w1070, "VISA resource name in"=w1071) -> ("error out"=w1074:errorcluster)  [unwired: 2 out]
            n667 = local write "Stage Moving"(TRUE ("Stage Moving")) -> ()
            n668 = local write "Stage Control Serial Error"(w1074) -> ()
          }
          frame #1 {
            n669 = local write "Stage Moving"(FALSE ("Stage Moving")) -> ()
            n670 = call <vilib>:"Beep.vi"() -> ()  [unwired: 3 in, 9 out]
          }
        }
      }
      event "Got ADig bead": Value Change {
        n671 = event-data() -> ()  [unwired: 1 in, 5 out]
        n672 = flat-sequence {
          frame #0 {
            n673 = local read "Cap 1 Samp Flow ON"() -> (w1085:bool)
            n674 = case shown="True" w1085 {
              frame False {
              }
              frame True {
                n675 = property on="Sample Channel\nFlow" class="Bool (strict)"("Val(Sgnl)"=TRUE ("Value (Signaling)")) -> ()  [unwired: 2 in, 2 out]
              }
            }
          }
          frame #1 {
            n676 = property on="Inject Pump 3" class="Bool (strict)"("Val(Sgnl)"=FALSE ("Value (Signaling)")) -> ()  [unwired: 2 in, 2 out]
          }
          frame #2 {
            n677 = property on="Move Cap. 1 (DNA Bottom)" class="Bool (strict)"("Val(Sgnl)"=TRUE ("Value (Signaling)")) -> ()  [unwired: 2 in, 2 out]
          }
        }
      }
      event "Force FB Data\nScript": Value Change {
        n678 = event-data() -> ()  [unwired: 1 in, 5 out]
        n679 = flat-sequence {
          tunnel: w1094 -> [w1098]
          tunnel: w1095 -> [w1099]
          tunnel: [w1099] -> w1090
          tunnel: [w1098] -> w1089
          tunnel: w1090 -> [w1102]
          tunnel: w1089 -> [w1101]
          tunnel: ["Trap Trig Fl."] -> w1091
          tunnel: [w1127] -> w1092
          tunnel: w1091 -> [w1127]
          tunnel: [w1131] -> w1093
          tunnel: w1092 -> [w1131]
          tunnel: w1093 -> [w1133]
          frame #0 {
            n680 = property on="Trap Delta (MHz)" class="DigNum (strict)"("Val(Sgnl)"="Trap Delta Before Moving") -> ()  [unwired: 2 in, 2 out]
          }
          frame #1 {
            n681 = local read "Saved Stage Positions"() -> (w1104:dbl[][])
            n682 = local write "FB Trap Pos Offset"(0.0 ("FB Trap Pos Offset")) -> ()
